vi "Read Tool Pose Data.vi"(8 "error in (no error)":errorcluster, 11 "UR5 Robot in":refnum<class "UR5 Robot.lvclass">) -> (0 "error out":errorcluster, 2 "Tool Pose Data":string, 3 "UR5 Robot out":refnum<class "UR5 Robot.lvclass">)   [LabVIEW 2018, in "UR5 Robot.lvlib" / "UR5 Robot.lvclass"]
uses:
  UR5 Robot.lvclass
  UR5 Robot.lvclass/UR5 Robot.ctl
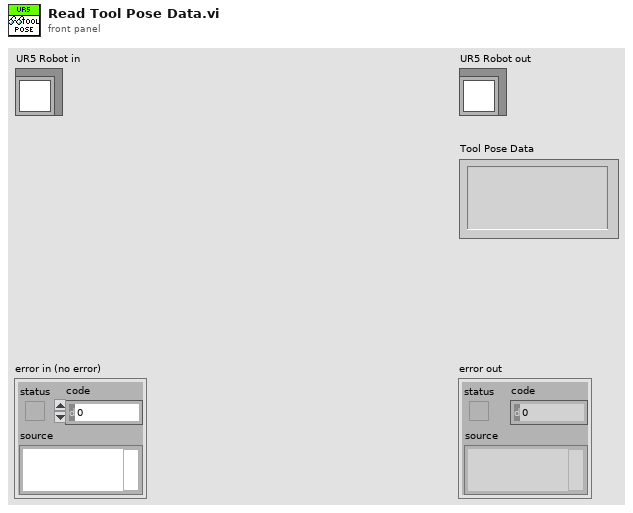
[diagram p1: front panel]
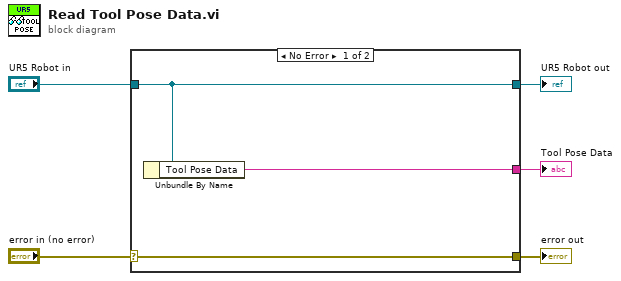
[diagram p0: block diagram]
diagram:
  n1 = case shown="No Error" "error in (no error)" {
    selector: "error in (no error)" -> [w8 w9]
    tunnel: [w8 w9] -> w4
    tunnel: [w7 w10] -> w2
    tunnel: "UR5 Robot in" -> [w7 w10]
    tunnel: [w6 _] -> w1
    frame No Error {
      n2 = Unbundle By Name(w7) -> ("Tool Pose Data"=w6:string)
    }
    frame Error {
    }
  }
  "error out" <- w4
  "UR5 Robot out" <- w2
  "Tool Pose Data" <- w1
